vi "Baseline_basic (SubVI).vi"(11 "S/g with baseline drift":dbl[](array[numeric])) -> (3 "Corrected":dbl[](array[numeric]))   [LabVIEW 2017]
uses:
  <vilib>/Analysis/NI_AALBase.lvlib
  <vilib>/Analysis/1siggen.llb/Ramp Pattern by Samples.vi
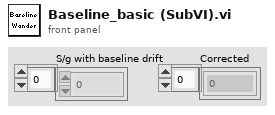
[diagram p1: front panel]
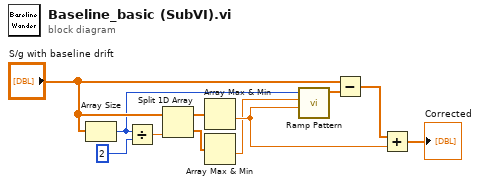
[diagram p0: block diagram]
diagram:
  n1 = Array Size(array="S/g with baseline drift") -> (size(s)=w8:i32)
  n2 = Divide(x=w8, y=2) -> (x/y=w7:dbl)
  n3 = Split 1D Array(array="S/g with baseline drift", index=w7) -> (first subarray=w2:dbl[], second subarray=w5:dbl[])
  n4 = Array Max & Min(array=w2) -> (min value=w9:dbl)  [unwired: 3 out]
  n5 = Array Max & Min(array=w5) -> (min value=w6:dbl)  [unwired: 3 out]
  n6 = call-poly <vilib>:"Ramp Pattern.vi"("start"=w9, "end"=w6, "samples"=w8) -> ("Ramp Pattern"=w3:dbl[])  [unwired: 7 in, 1 out]
  n7 = Subtract(x="S/g with baseline drift", y=w3) -> (x-y=w4:dbl[])
  n8 = Add(x=w4, y=w9) -> (x+y=→"Corrected":dbl[])
